vi "RSD Payload Parse.vi"(11 "Payload":string) -> (2 "Data (number)":i16[](array[numeric]), 3 "Data (string)":string[](array[string]))   [LabVIEW 2017, in "Samwontech TEMP2xxx.lvlib"]
uses:
  <instrlib>/Samwontech TEMP2xxx/Samwontech TEMP2xxx.lvlib
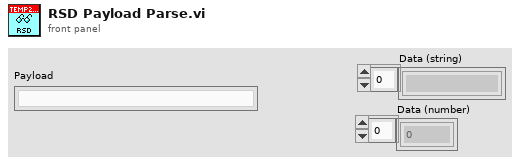
[diagram p1: front panel]
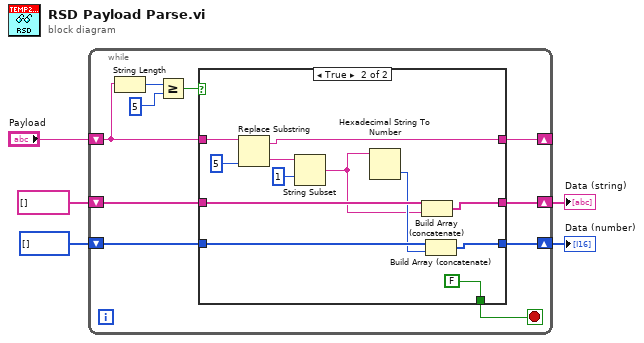
[diagram p0: block diagram]
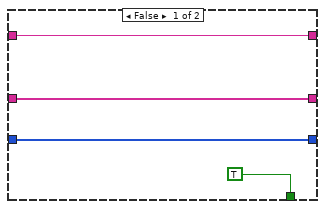
[diagram p2: hidden frame]
diagram:
  n1 = while {
    shift-right: [w6] -> _
    shift-left: "Payload" -> [w12]
    shift-right: [w9] -> w2
    shift-left: string[] [] -> [w11]
    shift-right: [w8] -> w1
    shift-left: u32[] [] -> [w10]
    stop <- w7 stop-if-true
    n2 = String Length(string=w12) -> (length=w15:i32)
    n3 = Greater Or Equal?(x=w15, y=5) -> (x >= y?=w13:bool)
    n4 = case shown="True" w13 {
      tunnel: w12 -> [w16 w25]
      tunnel: w11 -> [w19 w31]
      tunnel: w10 -> [w18 w29]
      tunnel: [w19 w30] -> w9
      tunnel: [w18 w27] -> w8
      tunnel: [TRUE FALSE] -> w7
      tunnel: [w16 w24] -> w6
      frame False {
      }
      frame True {
        n5 = Replace Substring(2:5 ("length (rest)"), 5:w25) -> (0:w22:string, 1:w24:string)  [unwired: 2 in]
        n6 = String Subset(string=w22, offset (0)=1) -> (substring=w20:string)  [unwired: 1 in]
        n7 = Hexadecimal String To Number(string=w20) -> (number=w28:u32)  [unwired: 2 in, 1 out]
        n8 = Build Array (concatenate)(w31, w20) -> (w30:string[])
        n9 = Build Array (concatenate)(w29, w28) -> (w27:u32[])
      }
    }
  }
  "Data (string)" <- w2
  "Data (number)" <- w1
